vi "GetNaturalDisplayOrientation.vi"(8 "No Error":errorcluster, 11 "Display ID":T2) -> (0 "Error Out":errorcluster, 3 "Display Orientation":T1)   [LabVIEW 2024, in "SDL3.lvlib" / "Video.lvlib"]
doc: "<B>Summary</B>\nGet the orientation of a display when it is unrotated."
uses:
  Video.lvlib
  DisplayID--integer.ctl
  DisplayOrientation--enum.ctl
  Lib/SDL3-32.dll
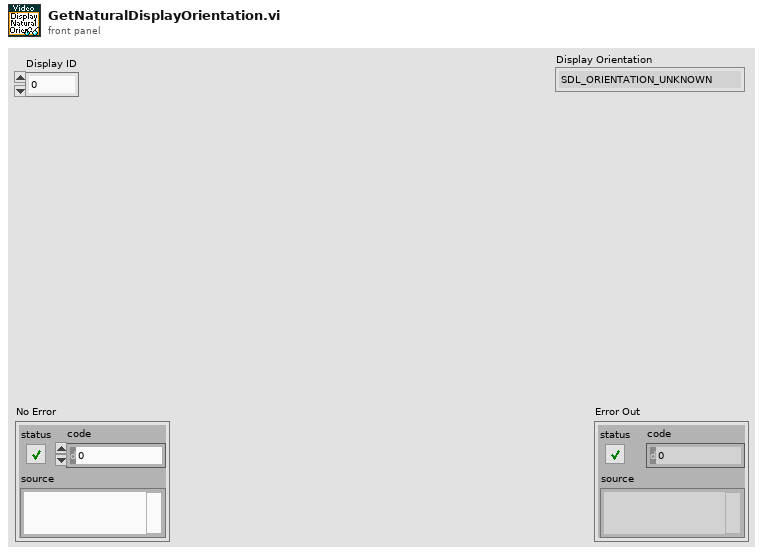
[diagram p1: front panel]
types:
  T1 = typedef "SDL3.lvlib/Video.lvlib/DisplayOrientation--enum.ctl" = enum32{"SDL_ORIENTATION_UNKNOWN", "SDL_ORIENTATION_LANDSCAPE", "SDL_ORIENTATION_LANDSCAPE_FLIPPED", "SDL_ORIENTATION_PORTRAIT", "SDL_ORIENTATION_PORTRAIT_FLIPPED"}
  T2 = typedef "SDL3.lvlib/Video.lvlib/DisplayID--integer.ctl" = u32
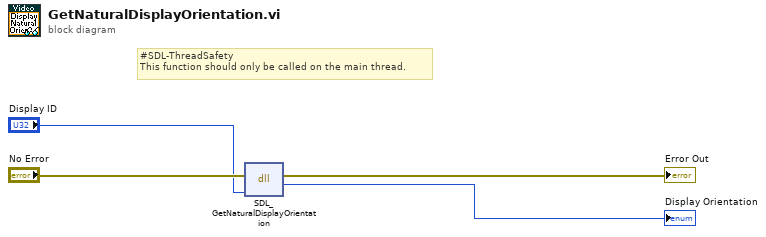
[diagram p0: block diagram]
diagram:
  # "#SDL-ThreadSafety\nThis function should only be called on the main thread."
  n1 = dll-call lib="C:/Users/Thomas/Documents/Projects/LV-SDL3/Lib/SDL3-*.*" fn="SDL_GetNaturalDisplayOrientation"(error in="No Error", "displayID"="Display ID") -> (error out=→"Error Out":errorcluster, "return type"=→"Display Orientation":u32)  [unwired: 3 in, 1 out]
